vi "DSP test 2.vi"() -> ()   [LabVIEW 2009, in "MicroDAQ.lvlib"]
uses:
  <instrlib>/MicroDAQ/MicroDAQ.lvlib
  <instrlib>/MicroDAQ/Channel/DSP/DSP.lvclass
  <instrlib>/MicroDAQ/MLink32.dll
panel:
  out "data out 2":dbl[][](array[numeric])
  in  "READ: Samples count 2":i32=1
  in  "XCOS SIGNAL ID 2":i32=2
  in  "Number of channels to read 2":i32=2
  in  "Rate [Hz]":dbl=10.0
  in  "stop":bool
  out "data out":dbl[][](array[numeric])
  in  "READ: Samples count":i32=1
  in  "XCOS SIGNAL ID":i32=1
  in  "Number of channels to read":i32=2
  in  "data in":sgl[](array[numeric])=[2.0, 3.0]
  in  "DSP binary path":path=path "C:/Program Files (x86)/National Instruments/LabVIEW 2014/instr.lib/MicroDAQ/Temp Tests/app2.out"
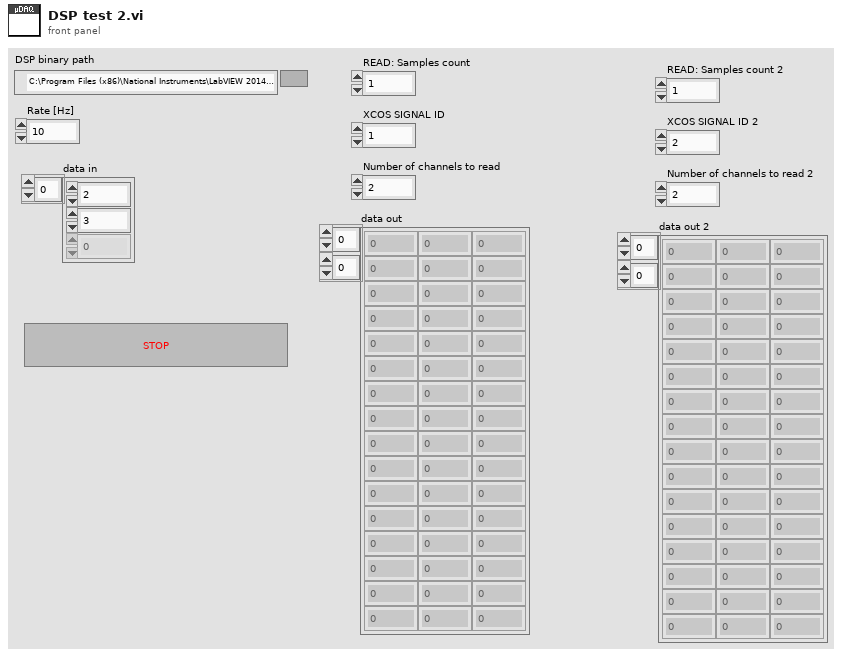
[diagram p1: front panel]
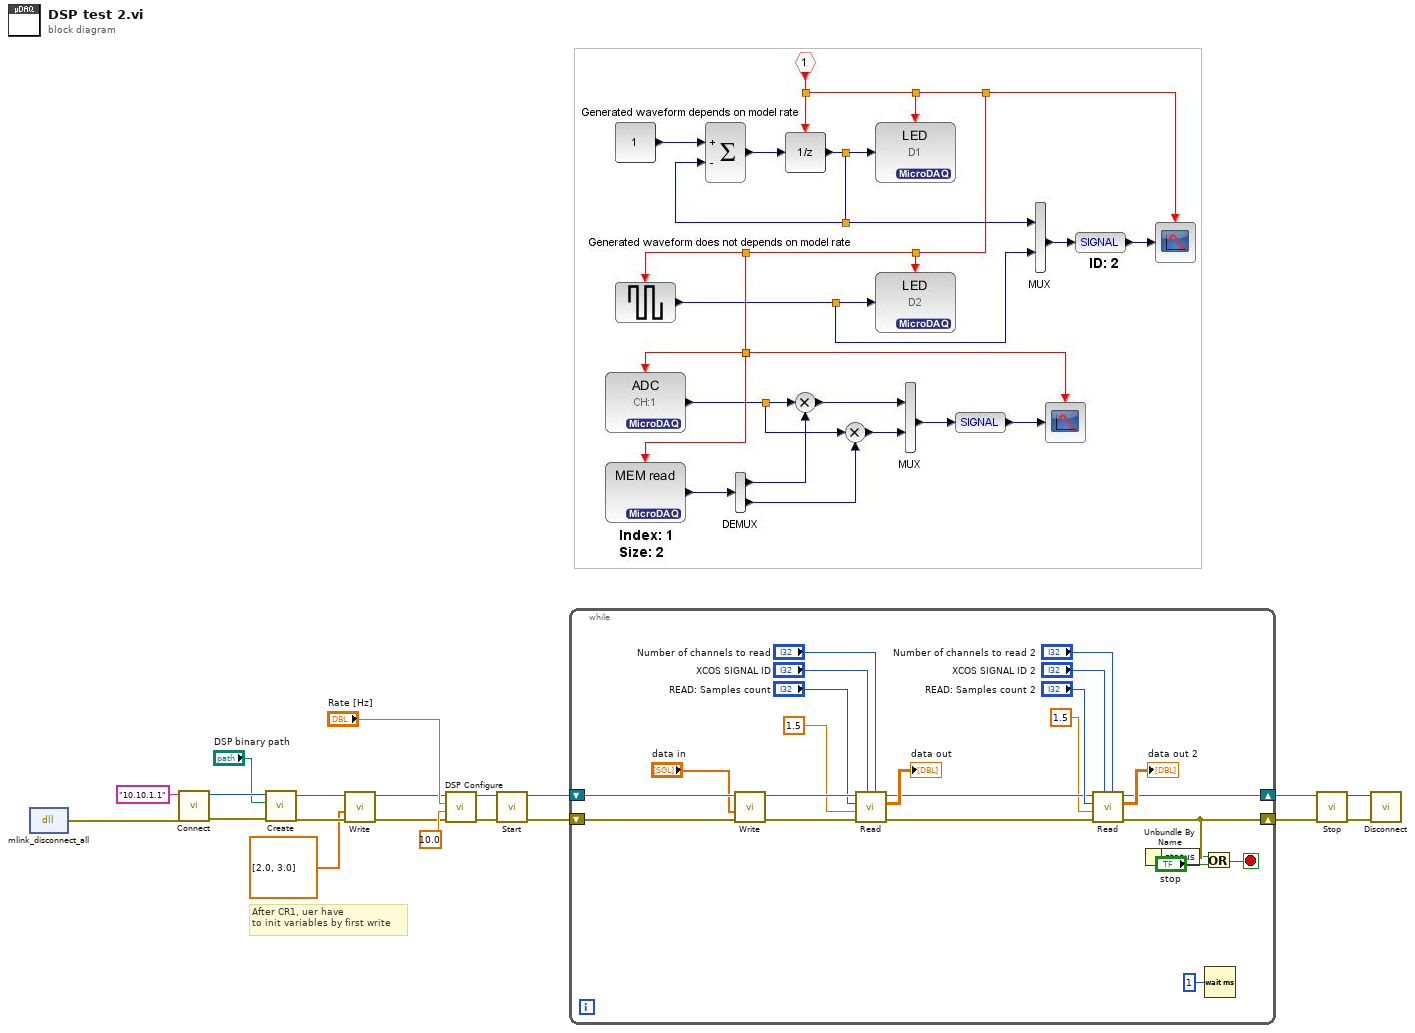
[diagram p0: block diagram]
diagram:
  # "After CR1, uer have\nto init variables by first write"
  n1 = dll-call lib="C:/Program Files (x86)/National Instruments/LabVIEW 2009/instr.lib/MicroDAQ/MLink32.dll" fn="mlink_disconnect_all" ("MLink32.*:mlink_connect")() -> (error out=w9:errorcluster)  [unwired: 4 in, 1 out]
  n2 = call <instrlib>:"Connect.vi"("error in (no error)"=w9, "IP address"="10.10.1.1") -> ("error out"=w19:errorcluster, "connection ID"=w18:i32)  [unwired: 8 in]
  n3 = call <instrlib>:"Create.vi"("error in (no error)"=w19, "DSP binary path"="DSP binary path", "connection ID"=w18) -> ("error out"=w4:errorcluster, "MicroDAQ.lvlib:DSP.lvclass"=w5:refnum<class "DSP.lvclass">)  [unwired: 7 in]
  n4 = call <instrlib>:"Write.vi"("error in"=w4, "data"=sgl[] [2.0, 3.0] ("Init Values"), "MicroDAQ.lvlib:DSP.lvclass"=w5) -> ("error out"=w2:errorcluster, "MicroDAQ.lvlib:DSP.lvclass out"=w3:refnum<class "DSP.lvclass">)  [unwired: 7 in]
  n5 = call <instrlib>:"DSP Configure.vi"("error in"=w2, "duration [s]"=10.0, "Rate [Hz]"="Rate [Hz]", "MicroDAQ.lvlib:DSP.lvclass"=w3) -> ("error out"=w8:errorcluster, "MicroDAQ.lvlib:DSP.lvclass out"=w11:refnum<class "DSP.lvclass">)  [unwired: 6 in]
  n6 = call-dynamic "Start.vi"("error in (no error)"=w8, "Task in"=w11) -> ("error out"=w7:errorcluster, "Task out"=w16:refnum<class "DSP.lvclass">)  [unwired: 8 in]
  n7 = while {
    shift-right: [w26] -> w14
    shift-left: w16 -> [w43]
    shift-right: [w25] -> w15
    shift-left: w7 -> [w34]
    stop <- w36 stop-if-true
    n8 = call <instrlib>:"Write.vi"("error in"=w34, "data"="data in", "MicroDAQ.lvlib:DSP.lvclass"=w43) -> ("error out"=w33:errorcluster, "MicroDAQ.lvlib:DSP.lvclass out"=w42:refnum<class "DSP.lvclass">)  [unwired: 7 in]
    n9 = call <instrlib>:"Read.vi"("Number of channels to read"="Number of channels to read", "signal id"="XCOS SIGNAL ID", "error in"=w33, "tiemout [s]"=1.5, "Samples count"="READ: Samples count", "MicroDAQ.lvlib:DSP.lvclass"=w42) -> ("error out"=w27:errorcluster, "data"=→"data out":dbl[][], "MicroDAQ.lvlib:DSP.lvclass out"=w28:refnum<class "DSP.lvclass">)  [unwired: 3 in]
    n10 = call <instrlib>:"Read.vi"("Number of channels to read"="Number of channels to read 2", "signal id"="XCOS SIGNAL ID 2", "error in"=w27, "tiemout [s]"=1.5, "Samples count"="READ: Samples count 2", "MicroDAQ.lvlib:DSP.lvclass"=w28) -> ("error out"=w25:errorcluster, "data"=→"data out 2":dbl[][], "MicroDAQ.lvlib:DSP.lvclass out"=w26:refnum<class "DSP.lvclass">)  [unwired: 3 in]
    n11 = Unbundle By Name(w25) -> ("status"=w23:bool)
    n12 = Or(x=w23, y="stop") -> (x .or. y?=w36:bool)
    n13 = Wait (ms)(milliseconds to wait=u32 1) -> ()  [unwired: 1 out]
  }
  n14 = call-dynamic "Stop.vi"("error in (no error)"=w15, "Task in"=w14) -> ("error out"=w13:errorcluster, "connection ID"=w12:i32)  [unwired: 8 in]
  n15 = call <instrlib>:"Disconnect.vi"("error in (no error)"=w13, "connection ID"=w12) -> ()  [unwired: 9 in, 1 out]
